vi "Read_PRINT_BT3564.vi"(8 "ERRIN":errorcluster caption="entrée d'erreur (pas d'erreur)", 10 "Arrêter":bool, 11 "VISA":refnum<visa-resource-name>) -> (0 "errout":errorcluster, 1 "Conti (Ohms)":dbl format="%#_10f", 2 "Conti (mOhms)":dbl format="%#_10f", 3 "DATA OUT":string)   [LabVIEW 2020]
uses:
  R_VG.vi
  OP300-ISO_SPI/SubVI/CONTI_END.vi
  <vilib>/Utility/inputDevices.llb/keyboardAcquire.vi
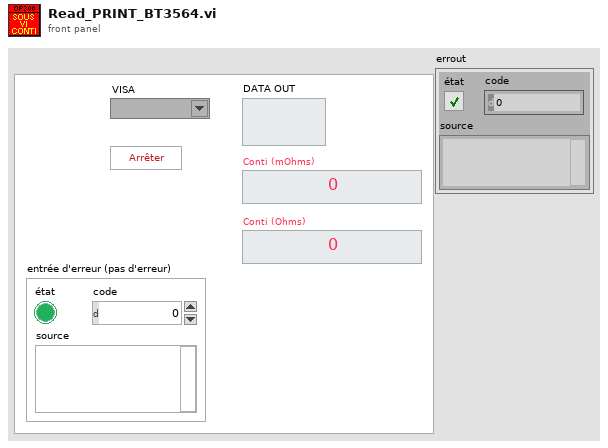
[diagram p1: front panel]
types:
  T1 = enum16{"0", "1", "2", "3", "4", "5", "6", "7", "8", "9", "A", "B", "C", "D", "E", "F", "G", "H", "I", "J", "K", "L", "M", "N", "O", "P", "Q", "R", "S", "T", "U", "V", "W", "X", "Y", "Z", "F1", "F2", "F3", "F4", "F5", "F6", "F7", "F8", "F9", "F10", "F11", "F12", "F13", "F14", "F15", "ADD", "BACK", "BACKSLASH", "CAPITAL", "COMMA", "DECIMAL", "DELETE", "DIVIDE", "DOWN", "END", "EQUALS", "ESCAPE", "GRAVE (`)", "HOME", "INSERT", "LBRACKET", "LCONTROL", "LEFT", "L ALT", "LSHIFT", "LWIN", "MINUS", "MULTIPLY", "NEXT", "NUMLOCK", "NUMPAD_0", "NUMPAD_1", "NUMPAD_2", "NUMPAD_3", "NUMPAD_4", "NUMPAD_5", "NUMPAD_6", "NUMPAD_7", "NUMPAD_8", "NUMPAD_9", "PAUSE", "PERIOD", "PRIOR (PG UP)", "RBRACKET", "RCONTROL", "RETURN", "RIGHT", "R ALT", "RSHIFT", "RWIN", "SCROLL", "SEMICOLON", "SLASH", "SPACE", "SUBTRACT", "TAB", "UP", "ENTER (num pad)", "' (quote)"}[]
  T2 = enum16{"0", "1", "2", "3", "4", "5", "6", "7", "8", "9", "A", "B", "C", "D", "E", "F", "G", "H", "I", "J", "K", "L", "M", "N", "O", "P", "Q", "R", "S", "T", "U", "V", "W", "X", "Y", "Z", "F1", "F2", "F3", "F4", "F5", "F6", "F7", "F8", "F9", "F10", "F11", "F12", "F13", "F14", "F15", "ADD", "BACK", "BACKSLASH", "CAPITAL", "COMMA", "DECIMAL", "DELETE", "DIVIDE", "DOWN", "END", "EQUALS", "ESCAPE", "GRAVE (`)", "HOME", "INSERT", "LBRACKET", "LCONTROL", "LEFT", "L ALT", "LSHIFT", "LWIN", "MINUS", "MULTIPLY", "NEXT", "NUMLOCK", "NUMPAD_0", "NUMPAD_1", "NUMPAD_2", "NUMPAD_3", "NUMPAD_4", "NUMPAD_5", "NUMPAD_6", "NUMPAD_7", "NUMPAD_8", "NUMPAD_9", "PAUSE", "PERIOD", "PRIOR (PG UP)", "RBRACKET", "RCONTROL", "RETURN", "RIGHT", "R ALT", "RSHIFT", "RWIN", "SCROLL", "SEMICOLON", "SLASH", "SPACE", "SUBTRACT", "TAB", "UP", "ENTER (num pad)", "' (quote)"}
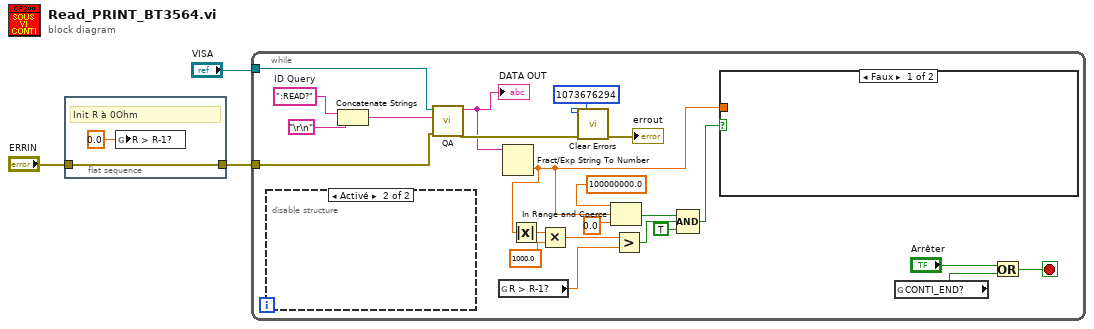
[diagram p0: block diagram]
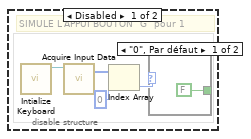
[diagram p2: hidden frame]
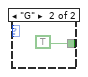
[diagram p3: hidden frame]
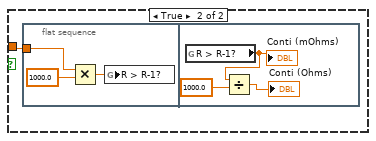
[diagram p4: hidden frame]
diagram:
  n1 = flat-sequence {
    tunnel: [w4] -> w1
    tunnel: "ERRIN" -> [w4]
    frame #0 {
      # "Init R à 0Ohm"
      n2 = global write "R_VG.vi" "R > R-1?"(0.0 ("R > R-1?")) -> ()
    }
  }
  n3 = while {
    tunnel: "VISA" -> [w24]
    tunnel: w1 -> [w10]
    stop <- w12 stop-if-true
    w28 = ":READ?"  # ID Query
    n4 = disable-structure shown="Activé" {
      frame Disabled {
        # "SIMULE L'APPUI BOUTON \"G\" pour 1"
        n5 = call <vilib>:"Intialize Keyboard.vi"() -> ("device ID"=w32:refnum<k1>)  [unwired: 10 in, 1 out]
        n6 = call-poly <vilib>:"Acquire Input Data.vi"("device ID"=w32) -> ("keys pressed"=w31:T1)  [unwired: 16 in, 2 out]
        n7 = Index Array(array=w31, index=0 ("indice")) -> (element=w29:T2)
        n8 = case shown="\"0\", Par défaut" w29 {
          tunnel: [FALSE TRUE] -> _
          frame "0", Default {
          }
          frame "G" {
          }
        }
      }
      frame Enabled {
      }
    }
    n9 = Concatenate Strings(w28, "\r\n") -> (w26:string)
    n10 = call "QA.vi"("ERRIN"=w10, "Chaîne"=w26, "VISA"=w24) -> ("ERROUT"=w27:errorcluster, "DATA OUT"=w8:string)  [unwired: 7 in]
    "DATA OUT" <- w8
    n11 = global read "R_VG.vi" "R > R-1?"() -> (w22:dbl)
    n12 = Fract/Exp String To Number(string=w8) -> (number=w14:dbl)  [unwired: 3 in, 1 out]
    n13 = Absolute Value(x=w14) -> (abs(x)=w7:dbl)
    n14 = Multiply(x=w7, y=1000.0) -> (x*y=w17:dbl)
    n15 = call <vilib>:"Clear Errors.vi"("error in (no error)"=w27, "specific error code to clear (0: all)"=1073676294) -> ("error out"=→"errout":errorcluster)  [unwired: 4 in, 1 out]
    n16 = In Range and Coerce(upper limit=100000000.0 ("limite supérieure"), x=w14, lower limit=0.0 ("limite inférieure")) -> (In Range?=w21:bool)  [unwired: 1 out]
    n17 = Greater?(x=w17, y=w22) -> (0:w20:bool)
    n18 = Compound Arithmetic op=AND ("Opérateur arithmétique")(w21, w20, TRUE ("valeur")) -> (w19:bool)
    n19 = case shown="Faux" w19 {
      tunnel: w14 -> [_ w35]
      frame False {
      }
      frame True {
        n20 = flat-sequence {
          tunnel: w35 -> [w37]
          frame #0 {
            n21 = Multiply(x=w37, y=1000.0) -> (x*y=w36:dbl)
            n22 = global write "R_VG.vi" "R > R-1?"(w36) -> ()
          }
          frame #1 {
            n23 = global read "R_VG.vi" "R > R-1?"() -> (w40:dbl)
            "Conti (mOhms)" <- w40
            n24 = Divide(x=w40, y=1000.0) -> (x/y=→"Conti (Ohms)":dbl)
          }
        }
      }
    }
    n25 = global read "CONTI_END.vi" "CONTI_END?"() -> (w9:bool)
    n26 = Or(x="Arrêter", y=w9) -> (x .or. y?=w12:bool)
  }
